vi "_Convert DAC to Mass.vi"(1 "Calibration Table":dbl[][](array[numeric]) format="%.2f", 2 "DAC":dbl format="%.2f") -> (0 "Mass":dbl format="%.2f")   [LabVIEW 2012]
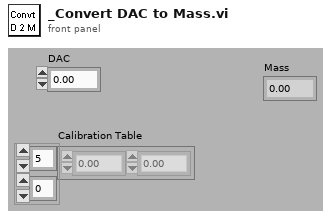
[diagram p1: front panel]
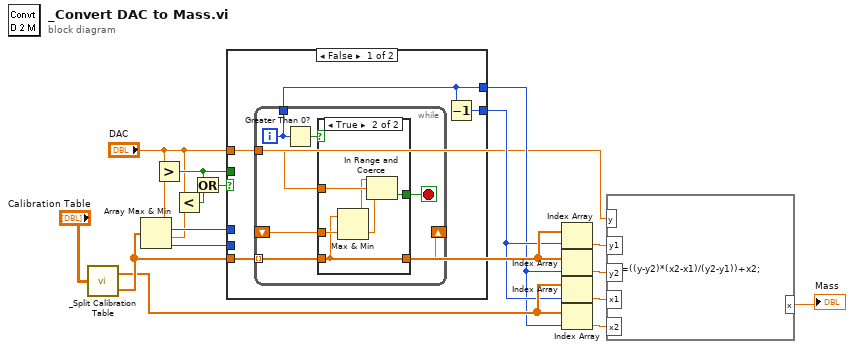
[diagram p0: block diagram]
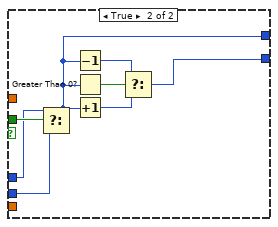
[diagram p3: hidden frame]
diagram:
  n1 = call "_Split Calibration Table.vi"("Calibration"="Calibration Table") -> ("Mass"=w9:dbl[], "DAC"=w10:dbl[])
  n2 = Array Max & Min(array=w10) -> (max value=w18:dbl, max index (indices)=w17:i32, min value=w13:dbl, min index (indices)=w12:i32)
  n3 = Greater?(x="DAC", y=w18) -> (0:w14:bool)
  n4 = Less?(x="DAC", y=w13) -> (x < y?=w16:bool)
  n5 = Or(x=w14, y=w16) -> (x .or. y?=w15:bool)
  n6 = case shown="False" w15 {
    tunnel: w10 -> [w22 _]
    tunnel: "DAC" -> [w21 _]
    tunnel: w17 -> [_ w43]
    tunnel: w14 -> [_ w44]
    tunnel: w12 -> [_ w42]
    tunnel: [w20 w39] -> w7
    tunnel: [w19 w37] -> w8
    frame False {
      n7 = while {
        tunnel: w22 -> [w29] mode=indexing
        tunnel: w21 -> [w25]
        shift-right: [w27] -> _
        shift-left: _ -> [w26]
        tunnel: [w23] -> w20
        i -> [w23]
        stop <- w24 stop-if-true
        n8 = Greater Than 0?(x=w23) -> (x > 0?=w28:bool)
        n9 = case shown="True" w28 {
          tunnel: w29 -> [w30 w35]
          tunnel: [w30 w35] -> w27
          tunnel: w26 -> [_ w36]
          tunnel: w25 -> [_ w34]
          tunnel: [_ w31] -> w24
          frame False {
          }
          frame True {
            n10 = Max & Min(x=w35, y=w36) -> (max(x,y)=w33:dbl, min(x,y)=w32:dbl)
            n11 = In Range and Coerce(upper limit=w33, x=w34, lower limit=w32) -> (In Range?=w31:bool)  [unwired: 1 out]
          }
        }
      }
      n12 = Decrement(x=w20) -> (x-1=w19:i32)
    }
    frame True {
      n13 = Select(t=w43, s=w44, f=w42) -> (s? t:f=w39:i32)
      n14 = Decrement(x=w39) -> (x-1=w40:i32)
      n15 = Greater Than 0?(x=w39) -> (x > 0?=w41:bool)
      n16 = Increment(x=w39) -> (x+1=w38:i32)
      n17 = Select(t=w40, s=w41, f=w38) -> (s? t:f=w37:i32)
    }
  }
  n18 = Index Array(array=w10, index=w8) -> (element=w6:dbl)
  n19 = Index Array(array=w10, index=w7) -> (element=w4:dbl)
  n20 = Index Array(array=w9, index=w8) -> (element=w3:dbl)
  n21 = Index Array(array=w9, index=w7) -> (element=w2:dbl)
  n22 = formula code="x=((y-y2)*(x2-x1)/(y2-y1))+x2;"("y1"=w6, "y2"=w4, "x1"=w3, "x2"=w2, "y"="DAC") -> ("x"=→"Mass":dbl)
